vi "commandTestAir.vi"(8 "error in (no error)":errorcluster, 10 "CommandTestAir in":T1, 11 "M1M3SAL in":refnum<class "M1M3SAL.lvclass">) -> (0 "error out":errorcluster, 2 "CommandTestAir out":T1, 3 "M1M3SAL out":refnum<class "M1M3SAL.lvclass">)   [LabVIEW 2016, in "M1M3SupportCommunicator.lvlib" / "M1M3SAL.lvclass"]
uses:
  M1M3SAL.lvclass
  DataTypes/Topics/CommandTestAir.ctl
  DataTypes/Topics/Parts/CommandId.ctl
  DataTypes/MessageHeader.ctl
  DataTypes/MessageTypes.ctl
  DataTypes/MessageTopics.ctl
  Common_RT_Utilities/U8ArrayBuilderAutoIndexing/U8ArrayBuilderAutoIndexing.lvclass
  M1M3SupportCommunicator.lvlib
  DataTypes/Topics/M1M3SupportTopics.lvlib
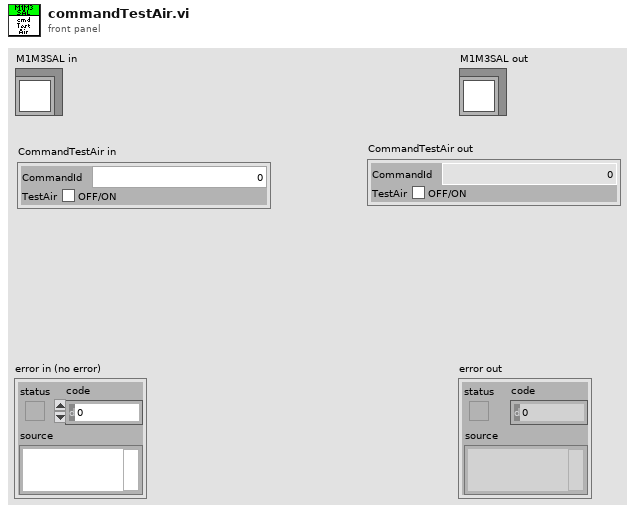
[diagram p1: front panel]
types:
  T1 = typedef "M1M3SupportTopics.lvlib/CommandTestAir.ctl" = cluster{"CommandId":T2, "TestAir":bool}
  T2 = typedef "M1M3SupportTopics.lvlib/CommandId.ctl" = i32
  T3 = typedef "M1M3SupportCommunicator.lvlib/MessageHeader.ctl" = cluster{"Type":T4, "Topic":T5, "Size":i32}
  T4 = typedef "M1M3SupportCommunicator.lvlib/MessageTypes.ctl" = enum8{"None", "PutSample", "GetNextSample", "LogEvent", "GetEvent", "IssueCommand", "CommandId", "WaitForCompletion", "AcceptCommand", "AckCommand"}
  T5 = typedef "M1M3SupportCommunicator.lvlib/MessageTopics.ctl" = enum8{"None", "ForceActuatorData", "MirrorForceData", "HardpointData", "AirData", "DynamicData", "FPGAData", "IMSData", "ForceActuatorStatus", "ElevationData", "HardpointStatus", "HardpointActuatorChase", "AirStatus", "ForceActuatorSafetyChecks", "ForceActuatorTest", "ActuatorBroadcastCounter", "StatusChecks", "CellChecks", "HardpointActuatorBreakaway", "RaiseMirrorComplete", "ILCCommunication", "ElevationAngleChecks", "DetailedState", "ServoLoops", "ForceActuatorInfo", "LowerMirrorComplete", "HardpointActuatorInfo", "SettingsApplied", "ErrorCode", "StartupChecks", "SummaryState", "SettingVersions", "ActuatorTestStatus", "AppliedSettingsMatchStart", "Enable", "EnterMaintenance", "Standby", "AbortLowerM1M3", "ApplyAberrationByForces", "ApplyAOSCorrectionByBendingModes", "ClearAOSCorrection", "Start", "RaiseM1M3", "TestForceActuator", "LowerM1M3", "ApplyAOSCorrectionByForces", "Disable", "ApplyAberationByBendingMode", "TestHardpoint", "ManipulateM1M3", "ClearAberration", "Exit", "TestAir", "AbortRaiseM1M3", "MoveHardpointActuators", "ExitMaintenance", "Shutdown"}
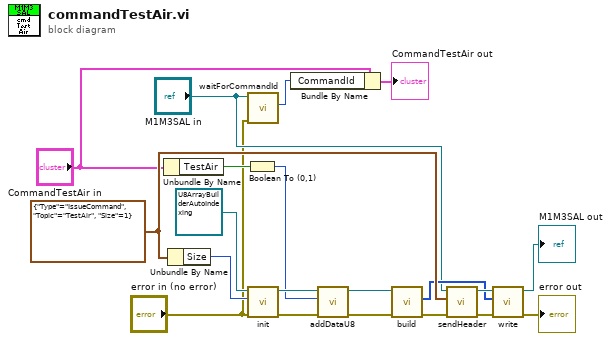
[diagram p0: block diagram]
diagram:
  w19 = T3 {"Type"=enum."IssueCommand", "Topic"=enum."TestAir", "Size"=1} ("MessageHeader")
  n1 = Unbundle By Name("CommandTestAir in") -> ("TestAir"=w15:bool)
  n2 = Unbundle By Name(w19) -> ("Size"=w18:i32)
  n3 = Boolean To (0,1)(Boolean=w15) -> (0, 1=w16:i16)
  n4 = call "waitForCommandId.vi"("error in (no error)"="error in (no error)", "M1M3SAL in"="M1M3SAL in") -> ("CommandId"=w7:T2)  [unwired: 7 in, 2 out]
  n5 = call "init.vi"("error in (no error)"="error in (no error)", "Size"=w18, "U8ArrayBuilderAutoIndexing in"=refnum<class "U8ArrayBuilderAutoIndexing.lvclass"> refnum ("RTUtilities.lvlib:U8ArrayBuilderAutoIndexing.lvclass")) -> ("error out"=w11:errorcluster, "U8ArrayBuilderAutoIndexing out"=w17:refnum<class "U8ArrayBuilderAutoIndexing.lvclass">)  [unwired: 7 in]
  n6 = Bundle By Name(cluster="CommandTestAir in", "CommandId"=w7) -> (→"CommandTestAir out":T1)
  n7 = call "addDataU8.vi"("error in (no error)"=w11, "Data"=w16, "U8ArrayBuilderAutoIndexing in"=w17) -> ("error out"=w10:errorcluster, "U8ArrayBuilderAutoIndexing out"=w14:refnum<class "U8ArrayBuilderAutoIndexing.lvclass">)  [unwired: 7 in]
  n8 = call "build.vi"("error in (no error)"=w10, "U8ArrayBuilderAutoIndexing in"=w14) -> ("error out"=w9:errorcluster, "Array"=w12:u8[])  [unwired: 7 in, 1 out]
  n9 = call "sendHeader.vi"("error in (no error)"=w9, "MessageHeader"=w19, "M1M3SAL in"="M1M3SAL in") -> ("error out"=w8:errorcluster, "M1M3SAL out"=w13:refnum<class "M1M3SAL.lvclass">)  [unwired: 7 in]
  n10 = call "write.vi"("error in (no error)"=w8, "Data"=w12, "M1M3SAL in"=w13) -> ("error out"=→"error out":errorcluster, "M1M3SAL out"=→"M1M3SAL out":refnum<class "M1M3SAL.lvclass">)  [unwired: 7 in]
